vi "CThread Terminal Node.vi"   [LabVIEW 2012, in "CThread.lvlib"]
uses:
  CThread.lvlib
  XNodes/terminalnode/CThread VI Terminal Node.xnode
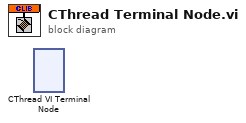
[diagram p0: block diagram]
diagram:
  n1 = xnode "CThread VI Terminal Node"() -> ()  [unwired: 1 in, 1 out]
